vi "Log STDs.vi"(8 "error in (no error)":errorcluster, 9 "StdErr":string, 10 "StdOut":string, 11 "Run Optimiser in":refnum<class "Optimiser Cell.lvclass">) -> (0 "error out":errorcluster, 3 "Run Optimiser out":refnum<class "Optimiser Cell.lvclass">)   [LabVIEW 2020, in "Run Utilities.lvlib" / "Optimiser Cell.lvclass"]
uses:
  Optimiser Cell.lvclass
  Optimiser Cell.lvclass/Optimiser Cell.ctl
  TALOS/TALOS_PPL.lvlibp/Classes/Log/Log.lvclass
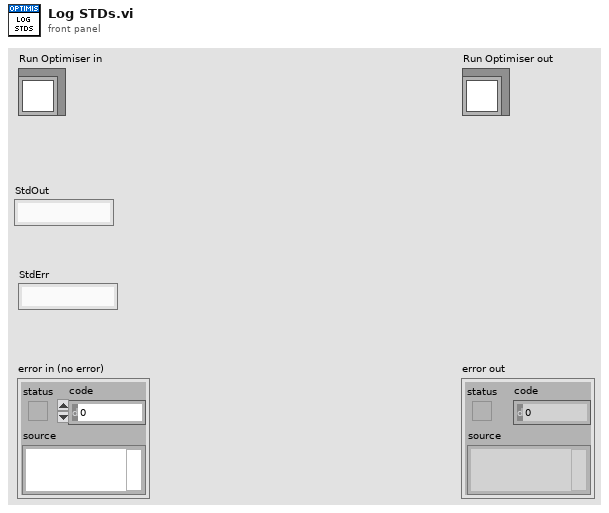
[diagram p1: front panel]
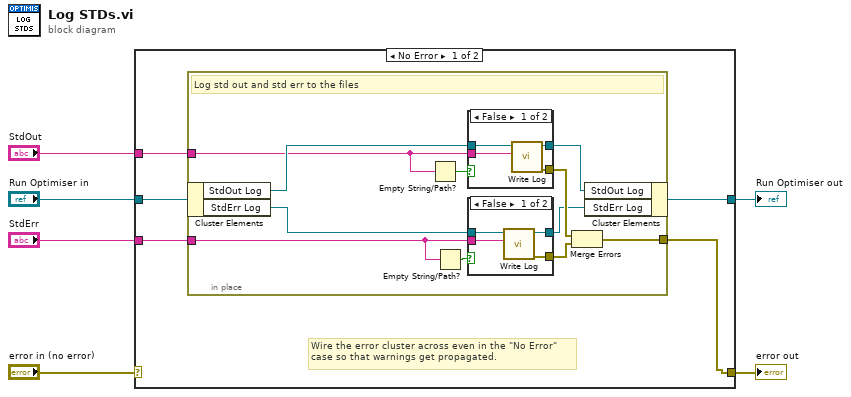
[diagram p0: block diagram]
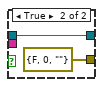
[diagram p2: hidden frame]
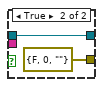
[diagram p3: hidden frame]
diagram:
  n1 = case shown="No Error" "error in (no error)" {
    selector: "error in (no error)" -> [_ w36]
    tunnel: [w9 w36] -> w5
    tunnel: [w10 w35] -> w3
    tunnel: "Run Optimiser in" -> [w11 w35]
    tunnel: "StdOut" -> [w8 _]
    tunnel: "StdErr" -> [w7 _]
    frame No Error {
      # "Wire the error cluster across even in the \"No Error\"\ncase so that warnings get propagated."
      n2 = in-place {
        in-place-border: [w14] -> w9
        in-place-border: w8 -> [w13]
        in-place-border: w7 -> [w12]
        # "Log std out and std err to the files"
        n3 = in-place-cluster #1(w11) -> ("StdOut Log"=w22:refnum<class "Log.lvclass">, "StdErr Log"=w17:refnum<class "Log.lvclass">)
        n4 = Empty String/Path?(string/path=w13) -> (empty?=w19:bool)
        n5 = Empty String/Path?(string/path=w12) -> (empty?=w16:bool)
        n6 = case shown="False" w19 {
          tunnel: w22 -> [w32 w34]
          tunnel: [w31 w34] -> w21
          tunnel: w13 -> [w30 _]
          tunnel: [w29 errorcluster {"status"=FALSE, "code"=0, "source"=""} ("error out")] -> w20
          frame False {
            n7 = call "Write Log.vi"("Text"=w30, "Log in"=w32) -> ("error out"=w29:errorcluster, "Log out"=w31:refnum<class "Log.lvclass">)  [unwired: 8 in]
          }
          frame True {
          }
        }
        n8 = case shown="False" w16 {
          tunnel: w17 -> [w26 w28]
          tunnel: [w25 w28] -> w15
          tunnel: w12 -> [w24 _]
          tunnel: [w23 errorcluster {"status"=FALSE, "code"=0, "source"=""} ("error out")] -> w18
          frame False {
            n9 = call "Write Log.vi"("Text"=w24, "Log in"=w26) -> ("error out"=w23:errorcluster, "Log out"=w25:refnum<class "Log.lvclass">)  [unwired: 8 in]
          }
          frame True {
          }
        }
        n10 = Merge Errors(w20, w18) -> (w14:errorcluster)
        n11 = in-place-cluster #1("StdOut Log"=w21, "StdErr Log"=w15) -> (w10:refnum<class "Optimiser Cell.lvclass">)
      }
    }
    frame Error {
    }
  }
  "error out" <- w5
  "Run Optimiser out" <- w3
